vi "WindDeltaVelocity.vi"(3 "Wind dV":dbl, 8 "Wind Velocity":dbl, 9 "Wind Direction":dbl, 10 "Robot Velocity":dbl, 11 "Robot Heading":dbl) -> ()   [LabVIEW 2012]
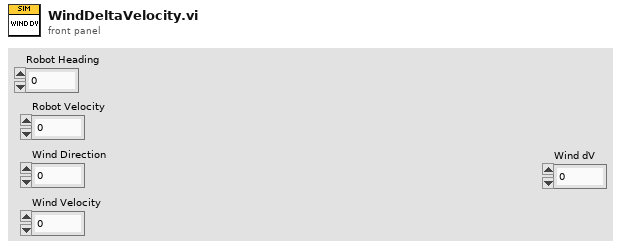
[diagram p1: front panel]
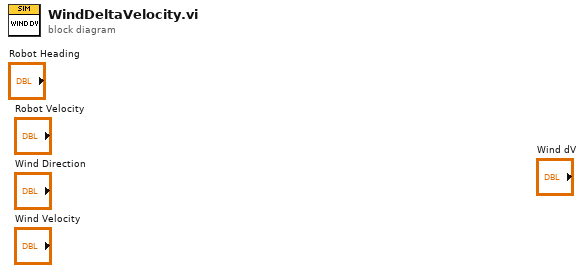
[diagram p0: block diagram]
diagram:
